vi "X509_NAME_get_string.vi"(8 "error in (no error)":errorcluster, 10 "X509_Name":u64, 11 "X509-Cert in":refnum<class "X509-Cert.lvclass">) -> (0 "error out":errorcluster, 2 "X509 Name String":string, 3 "X509-Cert out":refnum<class "X509-Cert.lvclass">)   [LabVIEW 2013, in "OpenSSL Socket.lvlib" / "X509-Cert.lvclass"]
uses:
  X509-Cert.lvclass
  SSL-Lib/SSL-Lib.lvclass/SSL-Lib.ctl
  BIO/BIO.lvclass/BIO.ctl
  SSL-Lib/Read Crypto Library Path.vi
  BIO/Read Handle.vi
  SSL-Lib/SSL-Lib.lvclass
  BIO/BIO.lvclass
panel:
  out "bytes written":i32
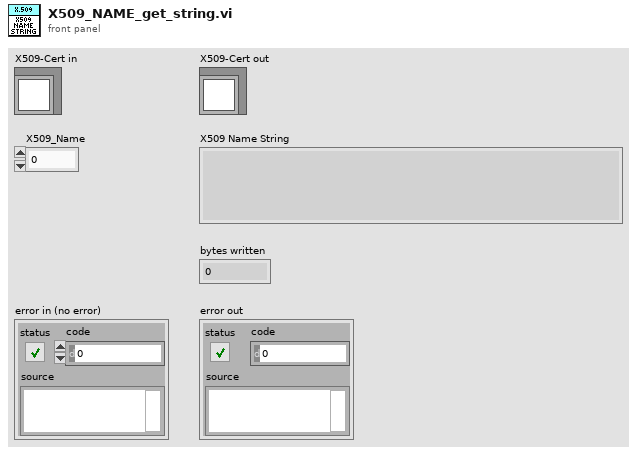
[diagram p1: front panel]
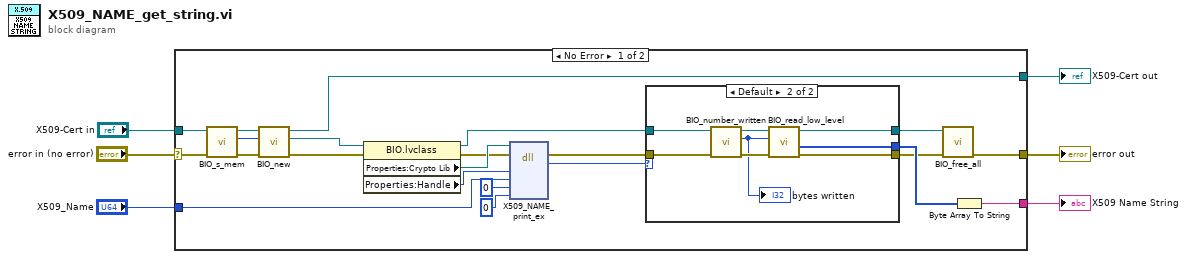
[diagram p0: block diagram]
diagram:
  n1 = case shown="No Error" "error in (no error)" {
    selector: "error in (no error)" -> [w11 w39]
    tunnel: "X509_Name" -> [w21 _]
    tunnel: [w7 _] -> w5
    tunnel: [w16 w39] -> w4
    tunnel: [w14 w40] -> w3
    tunnel: "X509-Cert in" -> [w13 w40]
    frame No Error {
      n2 = call "BIO_s_mem.vi"("error in (no error)"=w11, "SSL-Lib in"=w13) -> ("error out"=w8:errorcluster, "*BIO_Method"=w10:u64, "SSL-Lib out"=w9:refnum<class "X509-Cert.lvclass">)  [unwired: 7 in]
      n3 = call "BIO_new.vi"("error in (no error)"=w8, "*BIO_method"=w10, "SSL-Lib in"=w9) -> ("error out"=w18:errorcluster, "BIO out"=w25:refnum<class "BIO.lvclass">, "SSL-Lib out"=w14:refnum<class "X509-Cert.lvclass">)  [unwired: 6 in]
      n4 = property class="BIO.lvclass"(reference=w25, error in=w18) -> (reference out=w26:refnum<class "BIO.lvclass">, error out=w19:errorcluster, "Properties:Crypto Lib"=w28:path, "Properties:Handle"=w20:u64)
      n5 = dll-call lib="C:/Program Files (x86)/National Instruments/Shared/nissl/NIlibeay32.dll" fn="X509_NAME_print_ex"(path in=w28, error in=w19, "BIO"=w20, "X509_Name"=w21, "indent"=0, "flags"=u32 0) -> (error out=w24:errorcluster, "return type"=w27:i32)  [unwired: 5 in, 1 out]
      n6 = case shown="Default" w27 {
        tunnel: [w29 w36] -> w12
        tunnel: [w30 w34] -> w15
        tunnel: [_ w33] -> w17
        tunnel: w24 -> [w29 w32]
        tunnel: w26 -> [w30 w31]
        frame ..0 {
        }
        frame Default {
          n7 = call "BIO_number_written.vi"("error in (no error)"=w32, "BIO in"=w31) -> ("error out"=w38:errorcluster, "bytes written"=w37:i32, "BIO out"=w35:refnum<class "BIO.lvclass">)  [unwired: 7 in]
          "bytes written" <- w37
          n8 = call "BIO_read_low_level.vi"("error in (no error)"=w38, "bytes to read"=w37, "BIO in"=w35) -> ("error out"=w36:errorcluster, "buf"=w33:u8[], "BIO out"=w34:refnum<class "BIO.lvclass">)  [unwired: 5 in, 1 out]
        }
      }
      n9 = call "BIO_free_all.vi"("error in (no error)"=w12, "BIO in"=w15) -> ("error out"=w16:errorcluster)  [unwired: 9 in]
      n10 = Byte Array To String(unsigned byte array=w17) -> (string=w7:string)
    }
    frame Error {
    }
  }
  "X509 Name String" <- w5
  "error out" <- w4
  "X509-Cert out" <- w3
